vi "setTemperatureUnit.vi"(8 "error in (no error)":errorcluster, 10 "Temperature Unit (0: Celsius)":T1 items=["Celsius", "Fahrenheit", "Kelvin"], 11 "Electrometer in":refnum<class "Electrometer.lvclass">) -> (0 "error out":errorcluster, 3 "Electrometer out":refnum<class "Electrometer.lvclass">)   [LabVIEW 2016, in "Electrometer.lvclass"]
uses:
  Electrometer.lvclass
  TempUnits.ctl
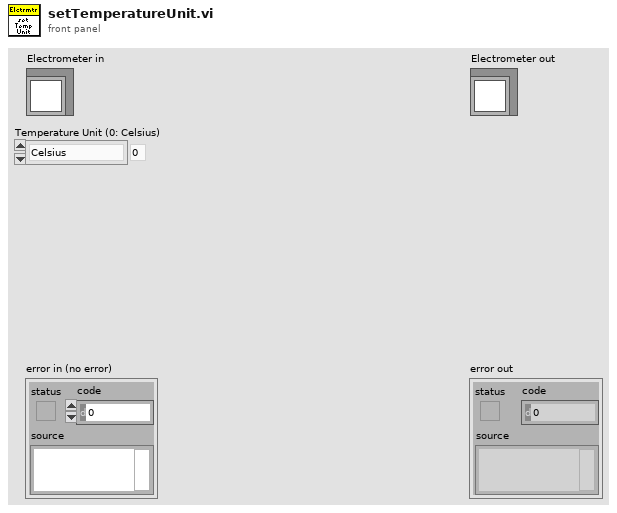
[diagram p1: front panel]
types:
  T1 = typedef "Electrometer.lvclass/TempUnits.ctl" = i32
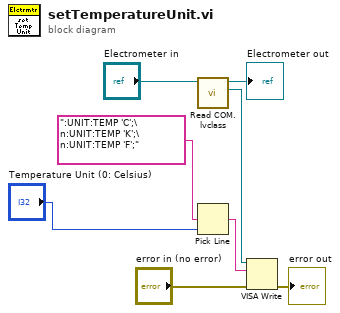
[diagram p0: block diagram]
diagram:
  n1 = call "Read COM.lvclass.vi"("Electrometer in"="Electrometer in") -> ("VISA"=w4:refnum<visa-resource-name>, "Electrometer out"=→"Electrometer out":refnum<class "Electrometer.lvclass">)  [unwired: 8 in, 1 out]
  n2 = Pick Line(multi-line string=":UNIT:TEMP 'C';\n:UNIT:TEMP 'K';\n:UNIT:TEMP 'F';", line index="Temperature Unit (0: Celsius)") -> (output string=w5:string)  [unwired: 1 in]
  n3 = VISA Write(VISA resource name=w4, write buffer=w5, error in (no error)="error in (no error)") -> (error out=→"error out":errorcluster)  [unwired: 2 out]
